vi "Stop Sweep Waveform.vi"(8 "error in (no error)":errorcluster, 10 "Waveforms in":waveform(dbl)[](array[waveform]), 11 "Generator in":refnum<class "Generator.lvclass">) -> (0 "error out":errorcluster, 2 "Waveforms out":waveform(dbl)[](array[waveform]), 3 "Generator out":refnum<class "Generator.lvclass">)   [LabVIEW 2019, in "Generator.lvclass"]
uses:
  Generator.lvclass
  Generator.lvclass/Generator.ctl
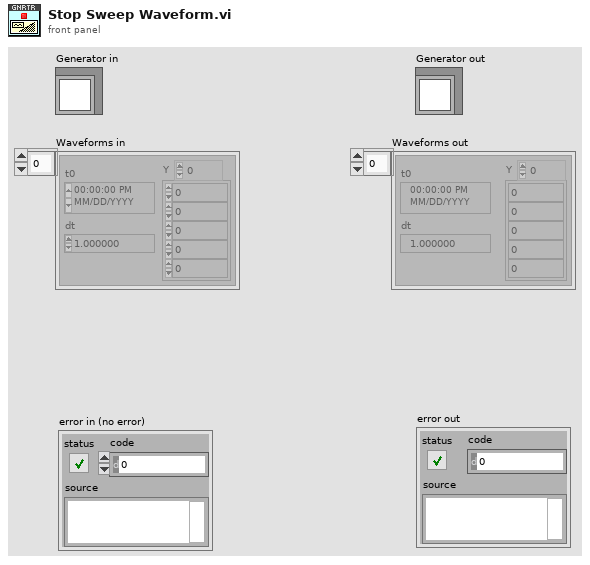
[diagram p1: front panel]
types:
  T1 = typedef "Generator.lvclass/Sweep.Channel--Cluster--Array.ctl" = T2[]
  T2 = typedef "Generator.lvclass/Sweep.Channel--Cluster.ctl" = cluster{"Enable?":bool, "Channel":u16, "Start":dbl, "End":dbl, "Pattern":T3, "Table":dbl[]}
  T3 = typedef "Generator.lvclass/Sweep.Pattern--Enum.ctl" = enum16{"Ramp /", "Ramp /\\", "Smooth Ramp _/", "Smooth Ramp _/\\_", "Table"}
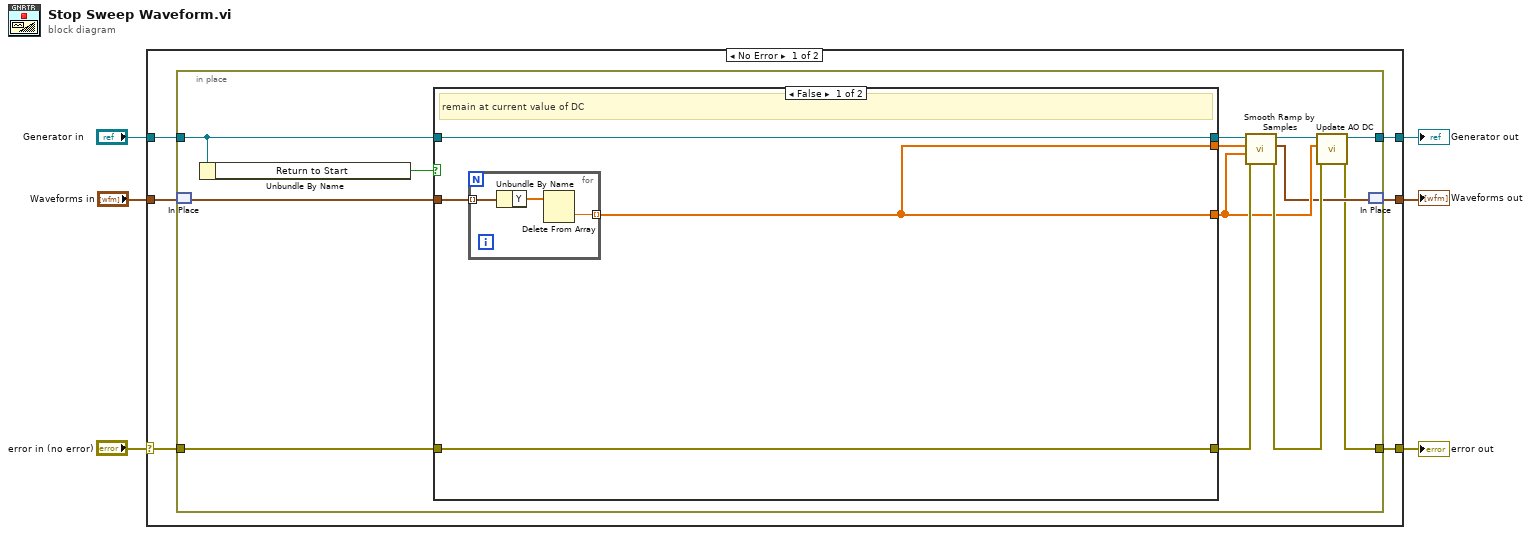
[diagram p0: block diagram]
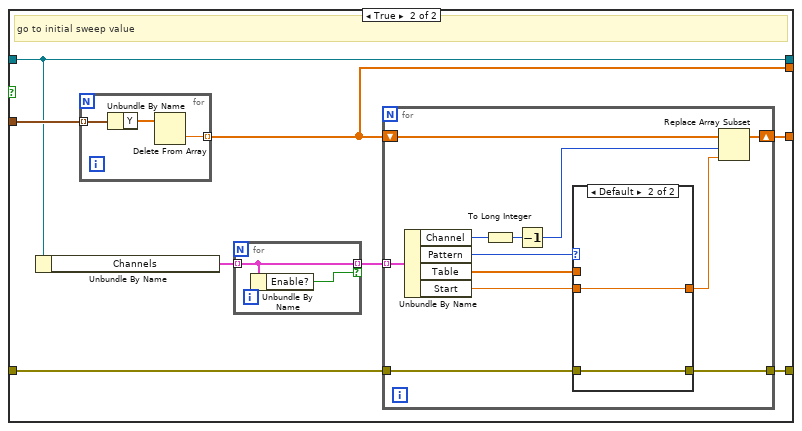
[diagram p2: hidden frame]
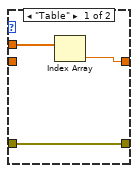
[diagram p3: hidden frame]
diagram:
  n1 = case shown="No Error" "error in (no error)" {
    selector: "error in (no error)" -> [w12 w64]
    tunnel: "Generator in" -> [w11 w63]
    tunnel: [w10 w63] -> w4
    tunnel: [w7 _] -> w3
    tunnel: [w9 w64] -> w2
    tunnel: "Waveforms in" -> [w8 _]
    frame No Error {
      n2 = in-place {
        in-place-border: w12 -> [w25]
        in-place-border: w11 -> [w23]
        in-place-border: [w14] -> w10
        in-place-border: [w13] -> w9
        n3 = in-place-match #1(w8) -> (w16:waveform(dbl)[])
        n4 = Unbundle By Name(w23) -> ("Return to Start"=w24:bool)
        n5 = case shown="False" w24 {
          tunnel: w25 -> [w28 w40]
          tunnel: [w28 w36] -> w19
          tunnel: w23 -> [w29 w35]
          tunnel: [w29 w35] -> w21
          tunnel: w16 -> [w27 w37]
          tunnel: [w26 w34] -> w18
          tunnel: [w26 w33] -> w17
          frame False {
            # "remain at current value of DC"
            n6 = for {
              tunnel: w27 -> [w32] mode=indexing
              tunnel: [w30] -> w26 mode=indexing
              n7 = Unbundle By Name(w32) -> ("Y"=w31:dbl[])
              n8 = Delete From Array(array=w31) -> (deleted portion=w30:dbl)  [unwired: 2 in, 1 out]
            }
          }
          frame True {
            # "go to initial sweep value"
            n9 = Unbundle By Name(w35) -> ("Channels"=w39:T1)
            n10 = for {
              tunnel: w37 -> [w43] mode=indexing
              tunnel: [w41] -> w34 mode=indexing
              n11 = Unbundle By Name(w43) -> ("Y"=w42:dbl[])
              n12 = Delete From Array(array=w42) -> (deleted portion=w41:dbl)  [unwired: 2 in, 1 out]
            }
            n13 = for {
              tunnel: w39 -> [w62] mode=indexing
              tunnel: [w62] -> w38 mode=indexing if=w61
              n14 = Unbundle By Name(w62) -> ("Enable?"=w61:bool)
            }
            n15 = for {
              tunnel: w38 -> [w52] mode=indexing
              tunnel: w40 -> [w55]
              tunnel: [w51] -> w36
              shift-right: [w45] -> w33
              shift-left: w34 -> [w44]
              n16 = Unbundle By Name(w52) -> ("Channel"=w53:u16, "Pattern"=w50:T3, "Table"=w49:dbl[], "Start"=w48:dbl)
              n17 = To Long Integer(number=w53) -> (32bit integer=w54:i32)
              n18 = Decrement(x=w54) -> (x-1=w47:i32)
              n19 = case shown="Default" w50 {
                tunnel: [w56 w59] -> w51
                tunnel: w55 -> [w56 w59]
                tunnel: w49 -> [w58 _]
                tunnel: w48 -> [_ w60]
                tunnel: [w57 w60] -> w46
                frame "Table" {
                  n20 = Index Array(array=w58) -> (element=w57:dbl)  [unwired: 1 in]
                }
                frame Default {
                }
              }
              n21 = Replace Array Subset(array=w44, new element=w46, index=w47) -> (w45:dbl[])
            }
          }
        }
        n22 = call "Smooth Ramp by Samples.vi"("error in (no error)"=w19, "End"=w17, "Start"=w18, "Generator in"=w21) -> ("Error out"=w20:errorcluster, "Waveforms out"=w15:waveform(dbl)[], "Generator out"=w22:refnum<class "Generator.lvclass">)  [unwired: 5 in]
        n23 = call "Update AO DC.vi"("error in (no error)"=w20, "AO.DC (V)"=w17, "Generator in"=w22) -> ("error out"=w13:errorcluster, "Generator out"=w14:refnum<class "Generator.lvclass">)  [unwired: 7 in]
        n24 = in-place-match #1(w15) -> (w7:waveform(dbl)[])
      }
    }
    frame Error {
    }
  }
  "error out" <- w2
  "Generator out" <- w4
  "Waveforms out" <- w3
